vi "Abort fgv.vi"(7 "Set?":bool, 11 "Value":bool) -> (3 "Value 2":bool)   [LabVIEW 2016]
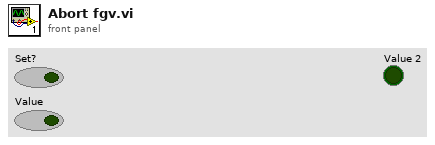
[diagram p1: front panel]
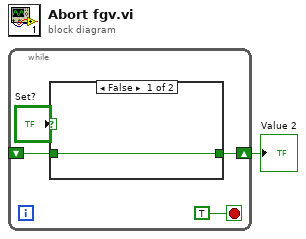
[diagram p0: block diagram]
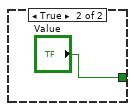
[diagram p2: hidden frame]
diagram:
  n1 = while {
    shift-right: [w3] -> w1
    shift-left: _ -> [w2]
    stop <- TRUE stop-if-true
    n2 = case shown="False" "Set?" {
      tunnel: [w6 "Value"] -> w3
      tunnel: w2 -> [w6 _]
      frame False {
      }
      frame True {
      }
    }
  }
  "Value 2" <- w1
